vi "Get variant DB to data.vi"(8 "error in (no error)":errorcluster, 11 "data in":variant[][](array[variant])) -> (0 "error out":errorcluster, 3 "data out":string[](array[string]))   [LabVIEW 2016]
doc: "Get variant to database! Extract 2D array data into 1D array data."
uses:
  <vilib>/addons/database/_DB Variant To Data/Database Variant To Data.xnode
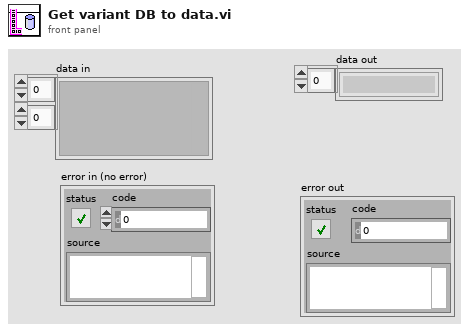
[diagram p1: front panel]
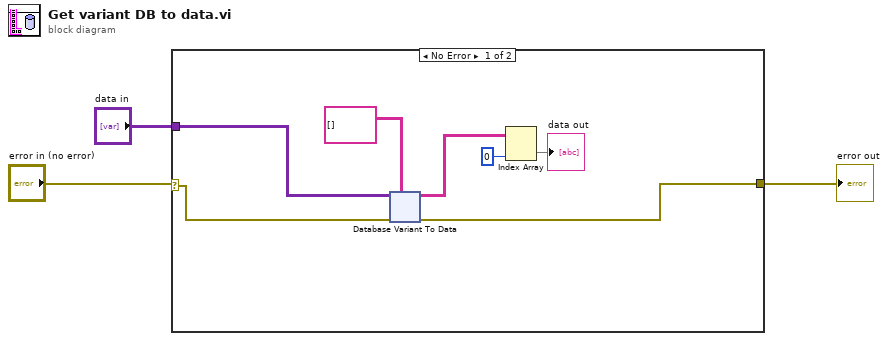
[diagram p0: block diagram]
diagram:
  n1 = case shown="No Error" "error in (no error)" {
    selector: "error in (no error)" -> [w6 w55]
    tunnel: [w5 w55] -> w2
    tunnel: "data in" -> [w4 _]
    frame No Error {
      n2 = xnode "Database Variant To Data"("database variant"=w4, "error in (no error)"=w6, "type"=string[][] [] ("Array")) -> ("data"=w9:string[][], "error out"=w5:errorcluster)
      n3 = Index Array(array=w9, index (col)=0 ("disabled index (col)")) -> (element=→"data out":string[])  [unwired: 1 in]
    }
    frame Error {
    }
  }
  "error out" <- w2
